vi "NetSlopeDetect.vi"(9 "SigInput":i16[](array[numeric]), 10 "+/- Slope":bool, 11 "On/Off":bool) -> (3 "Boolean":bool)   [LabVIEW 2018]
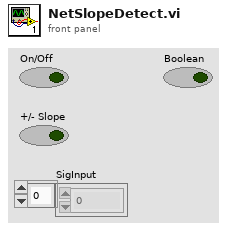
[diagram p1: front panel]
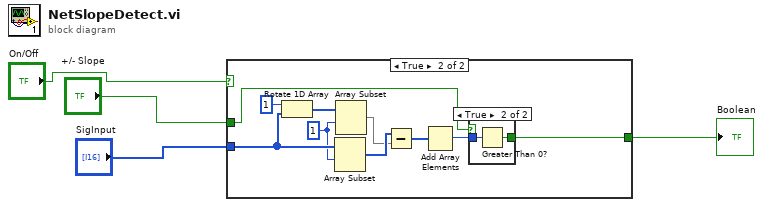
[diagram p0: block diagram]
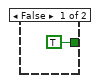
[diagram p2: hidden frame]
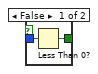
[diagram p3: hidden frame]
diagram:
  n1 = case shown="True" "On/Off" {
    tunnel: "SigInput" -> [_ w13]
    tunnel: [TRUE w7] -> w4
    tunnel: "+/- Slope" -> [_ w6]
    frame False {
    }
    frame True {
      w12 = 1 ("index")
      n2 = Rotate 1D Array(1:w13, 2:1 ("n")) -> (0:w14:i16[])
      n3 = Array Subset(array=w13, index=w12) -> (w11:i16[])  [unwired: 1 in]
      n4 = Array Subset(array=w14, index=w12) -> (w10:i16[])  [unwired: 1 in]
      n5 = Subtract(x=w11, y=w10) -> (x-y=w9:i16[])
      n6 = Add Array Elements(numeric array=w9) -> (sum=w8:i16)
      n7 = case shown="True" w6 {
        tunnel: w8 -> [w16 w19]
        tunnel: [w17 w18] -> w7
        frame False {
          n8 = Less Than 0?(x=w16) -> (x < 0?=w17:bool)
        }
        frame True {
          n9 = Greater Than 0?(x=w19) -> (x > 0?=w18:bool)
        }
      }
    }
  }
  "Boolean" <- w4
